vi "U8toHEX.vi"(11 "data":u8) -> (3 "HEX":string)   [LabVIEW 2018]
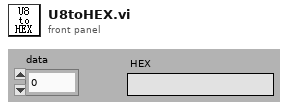
[diagram p1: front panel]
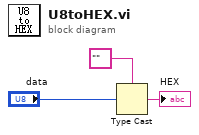
[diagram p0: block diagram]
diagram:
  n1 = Type Cast(type="", x="data") -> (*(type *) &x=→"HEX":string)
